vi "NextRecordFocus2DListCtrl.vi"(11 "multiple list in":refnum<vi>) -> (2 "is empty?":bool, 3 "multiple list out":refnum<vi>)   [LabVIEW 2018, in "Library-Ctrl.lvlib"]
uses:
  Library-Ctrl.lvlib
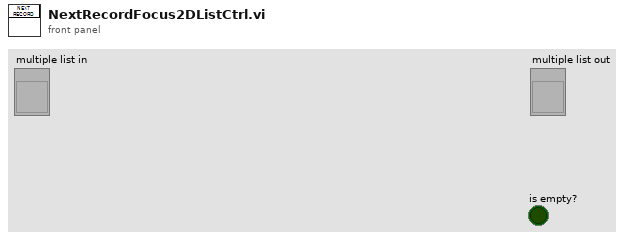
[diagram p1: front panel]
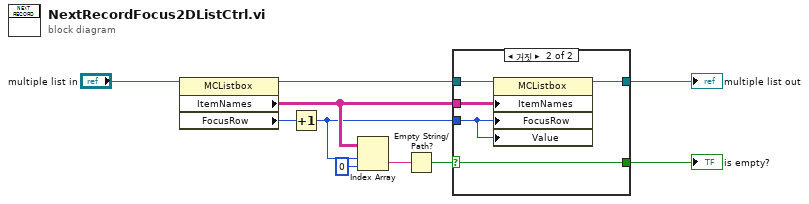
[diagram p0: block diagram]
diagram:
  n1 = property class="MCListbox"(reference="multiple list in") -> (reference out=w8:refnum<vi>, "ItemNames"=w6:string[][], "FocusRow"=w10:i32)  [unwired: 1 in, 1 out]
  n2 = Increment(x=w10) -> (x+1=w5:i32)
  n3 = Index Array(array=w6, index (row)=w5, index (col)=0 ("비활성화된 인덱스 (열)")) -> (element=w3:string)
  n4 = Empty String/Path?(string/path=w3) -> (empty?=w2:bool)
  n5 = case shown="거짓" w2 {
    selector: w2 -> [w11 w13]
    tunnel: w8 -> [w12 w17]
    tunnel: [w12 w16] -> w7
    tunnel: w6 -> [_ w15]
    tunnel: w5 -> [_ w14]
    tunnel: [w11 w13] -> w1
    frame True {
    }
    frame False {
      n6 = property class="MCListbox"(reference=w17, "ItemNames"=w15, "FocusRow"=w14, "Value"=w14) -> (reference out=w16:refnum<vi>)  [unwired: 1 in, 1 out]
    }
  }
  "multiple list out" <- w7
  "is empty?" <- w1
